vi "Engine Out - Port Fuel Injectors.vi"(0 "PFI Quantities [mg/inj]":sgl[](array[numeric]), 1 "PFI Timings [DBTDC]":sgl[](array[numeric]), 2 "BattV [V]":sgl, 5 "Control Inputs":T2={"Engine Speed [RPM]"=0.0, "Engine Status"=enum."STALLED", "Load Control \nMode"=enum."High-Idle Governor", "dt(s)"=0.0, "Number of Cylinders"=0, "Engine Displacement [cc]"=0.0, "StoichAFR"=0.0, "Q.LHV Fuel [kJ/kg]"=0.0, "BattV PSU [V]"=0.0, "12V PSU [V]"=0.0, "5V PSU [V]"=0.0, "Pedal Position [%]"=0.0, "Oil Pressure [kPa]"=0.0, "Oil Temp [C]"=0.0, "Oil Level [%]"=0.0, "Engine Coolant Temp (ECT) [C]"=0.0, "Engine Coolant Pressure [kPa]"=0.0, "Rail Pressure [bar]"=0.0, "Fuel Pressure [kPa]"=0.0, "Fuel Temp [C]"=0.0, "Vacuum Pressure [kPa]"=0.0, "Throttle Position [%]"=0.0, "Cam1 Advance [CAD]"=0.0, "Cam2 Advance [CAD]"=0.0, "Cam3 Advance [CAD]"=0.0, "Cam4 Advance [CAD]"=0.0, "CA50 Control Output [CAD]"=[], "CA50 Control Output Valid"=[], "Intake Air Temp (IAT) [C]"=0.0, "Barometric Air Pressure [kPa]"=0.0, "Intake Air Rel. Humidity [%]"=0.0, "Mass Air Flow (MAF) [kg/hr]"=0.0, "Turbo Inlet Air Pressure [kPa]"=0.0, "Turbo Inlet Air Temp [C]"=0.0, "Turbo Outlet Air Pressure [kPa]"=0.0, "Turbo Outlet Air Temp [C]"=0.0, "CAC Outlet Pressure [kPa]"=0.0, "CAC Outlet Temp [C]"=0.0, "Intake Manifold Pressure (MAP) [kPa]"=0.0, "Intake Manifold Temp (MAT) [C]"=0.0, "Exhaust Manifold Pressure [kPa]"=0.0, "Exhaust Manifold Temp [C]"=0.0, "HighP EGR Cooler Outlet Pressure [kPa]"=0.0, "HighP EGR Cooler Outlet Temp [C]"=0.0, "HighP EGR Differential Pressure [kPa]"=0.0, "HighP EGR Valve Position [%]"=0.0, "Turbo Outlet Exhaust Pressure [kPa]"=0.0, "Turbo Outlet Exhaust Temp [C]"=0.0, "VGT Position 1 [%]"=0.0, "VGT Position 2 [%]"=0.0, "Turbo Speed 1 [RPM]"=0.0, "Turbo Speed 2 [RPM]"=0.0, "LowP EGR Differential Pressure [kPa]"=0.0, "LowP EGR Valve Position [%]"=0.0, "UEGO1Lambda"=0.0, "UEGO1_Hot"=FALSE, "UEGO2Lambda"=0.0, "UEGO2_Hot"=FALSE, "Knock Intensity"=[], "Knock"=[]} {"Knock Intensity" format="%.2f"; "CA50 Control Output [CAD]" format="%.2f"; "Exhaust Manifold Temp [C]" format="%#_6f"; "UEGO2Lambda" format="%.2f"; "Intake Manifold Temp (MAT) [C]" format="%#_6f"; "UEGO1Lambda" format="%.2f"}) -> (11 "Injector 8":T1, 13 "Injector 7":T1, 14 "Injector 1":T1, 15 "Injector 2":T1, 16 "Injector 3":T1, 17 "Injector 4":T1, 18 "Injector 5":T1, 19 "Injector 6":T1)   [LabVIEW 2015, in "ECS-RT.lvlib"]
uses:
  ECS-RT.lvlib
  Typedefs/Control Inputs/Control Inputs.ctl
  Typedefs/EPT/Engine Status.ctl
  Typedefs/MISC/Load Control Mode.ctl
  Typedefs/Raw Outputs/PFI.ctl
  ECS-Shared.lvlib
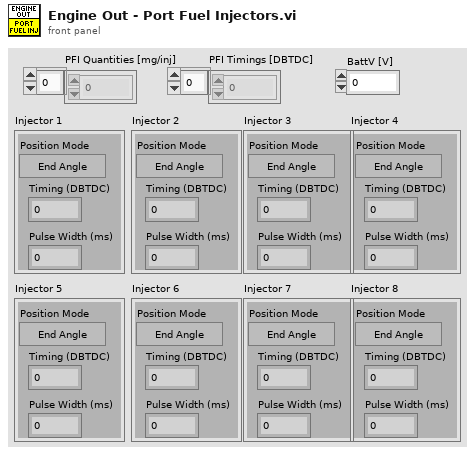
[diagram p1: front panel]
types:
  T1 = typedef "ECS-Shared.lvlib/PFI.ctl" = cluster{"Position Mode":bool, "Timing (DBTDC)":sgl, "Pulse Width (ms)":sgl}
  T2 = typedef "ECS-Shared.lvlib/Control Inputs.ctl" = cluster{"Engine Speed [RPM]":sgl, "Engine Status":T3, "Load Control \nMode":T4, "dt(s)":sgl, "Number of Cylinders":u8, "Engine Displacement [cc]":sgl, "StoichAFR":sgl, "Q.LHV Fuel [kJ/kg]":sgl, "BattV PSU [V]":sgl, "12V PSU [V]":sgl, "5V PSU [V]":sgl, "Pedal Position [%]":sgl, "Oil Pressure [kPa]":sgl, "Oil Temp [C]":sgl, "Oil Level [%]":sgl, "Engine Coolant Temp (ECT) [C]":sgl, "Engine Coolant Pressure [kPa]":sgl, "Rail Pressure [bar]":sgl, "Fuel Pressure [kPa]":sgl, "Fuel Temp [C]":sgl, "Vacuum Pressure [kPa]":sgl, "Throttle Position [%]":sgl, "Cam1 Advance [CAD]":sgl, "Cam2 Advance [CAD]":sgl, "Cam3 Advance [CAD]":sgl, "Cam4 Advance [CAD]":sgl, "CA50 Control Output [CAD]":sgl[], "CA50 Control Output Valid":bool[], "Intake Air Temp (IAT) [C]":sgl, "Barometric Air Pressure [kPa]":sgl, "Intake Air Rel. Humidity [%]":sgl, "Mass Air Flow (MAF) [kg/hr]":sgl, "Turbo Inlet Air Pressure [kPa]":sgl, "Turbo Inlet Air Temp [C]":sgl, "Turbo Outlet Air Pressure [kPa]":sgl, "Turbo Outlet Air Temp [C]":sgl, "CAC Outlet Pressure [kPa]":sgl, "CAC Outlet Temp [C]":sgl, "Intake Manifold Pressure (MAP) [kPa]":sgl, "Intake Manifold Temp (MAT) [C]":sgl, "Exhaust Manifold Pressure [kPa]":sgl, "Exhaust Manifold Temp [C]":sgl, "HighP EGR Cooler Outlet Pressure [kPa]":sgl, "HighP EGR Cooler Outlet Temp [C]":sgl, "HighP EGR Differential Pressure [kPa]":sgl, "HighP EGR Valve Position [%]":sgl, "Turbo Outlet Exhaust Pressure [kPa]":sgl, "Turbo Outlet Exhaust Temp [C]":sgl, "VGT Position 1 [%]":sgl, "VGT Position 2 [%]":sgl, "Turbo Speed 1 [RPM]":sgl, "Turbo Speed 2 [RPM]":sgl, "LowP EGR Differential Pressure [kPa]":sgl, "LowP EGR Valve Position [%]":sgl, "UEGO1Lambda":sgl, "UEGO1_Hot":bool, "UEGO2Lambda":sgl, "UEGO2_Hot":bool, "Knock Intensity":sgl[], "Knock":bool[]}
  T3 = typedef "ECS-Shared.lvlib/Engine Status.ctl" = enum16{"OFF", "STALLED", "CRANKING", "RUNNING", "ACCEL", "DECEL", "SAFE"}
  T4 = typedef "ECS-Shared.lvlib/Load Control Mode.ctl" = enum16{"No Governor", "Low-Idle Governor", "High-Idle Governor"}
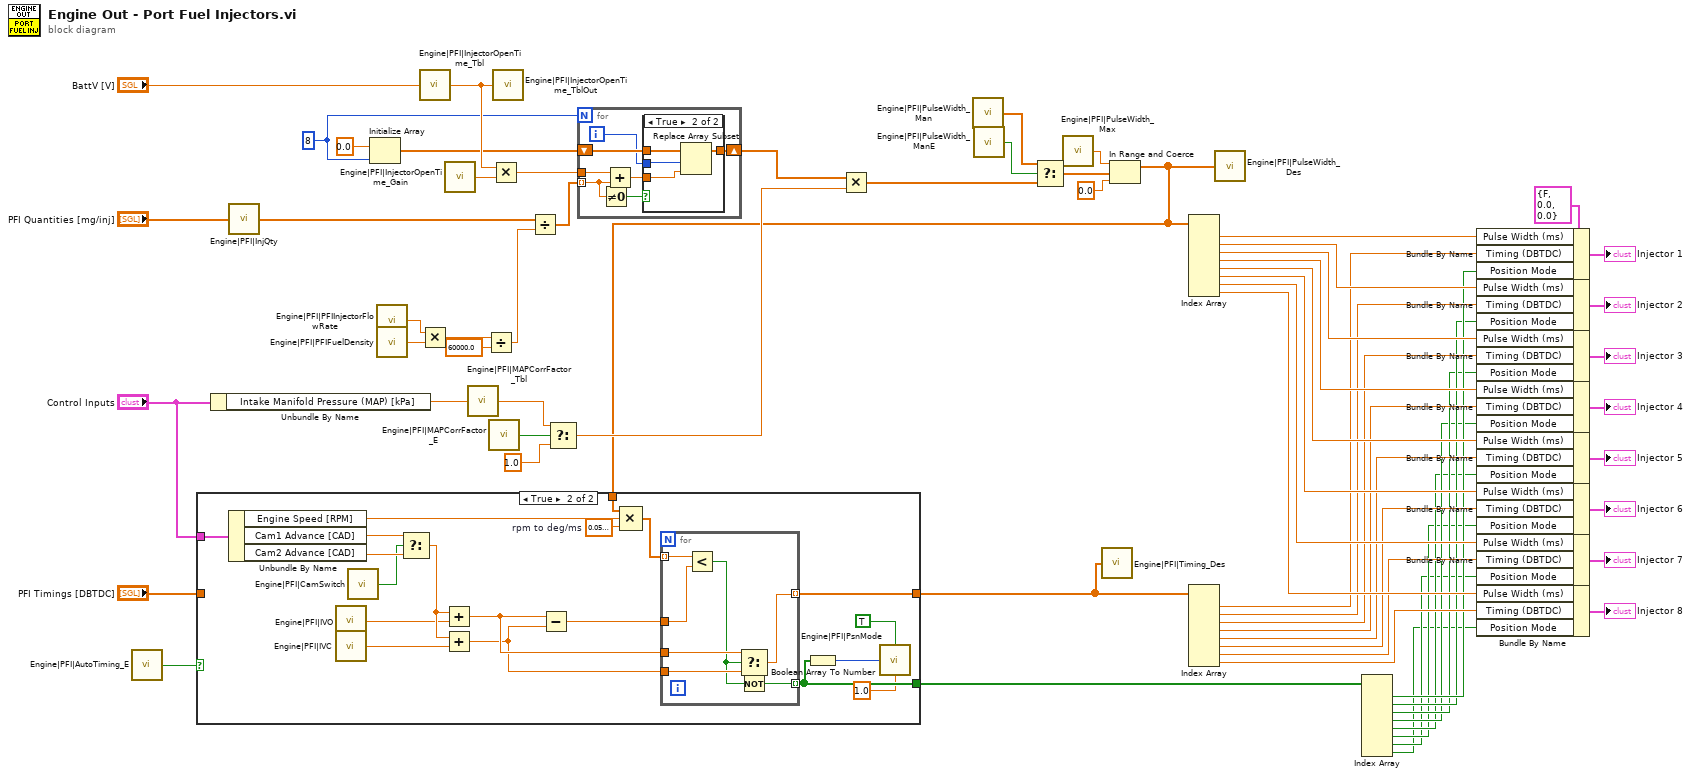
[diagram p0: block diagram]
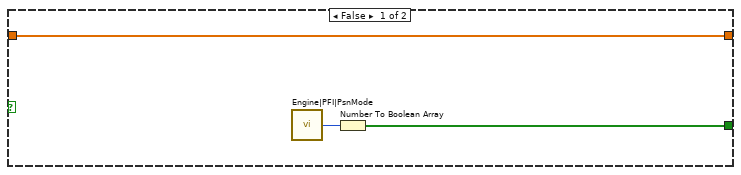
[diagram p3: hidden frame]
diagram:
  w1 = 8 ("dimension size")
  w43 = T1 {"Position Mode"=FALSE, "Timing (DBTDC)"=0.0, "Pulse Width (ms)"=0.0} ("Injector")
  n1 = call "Engine|PFI|AutoTiming_E"() -> ("Value"=w11:bool)
  n2 = Unbundle By Name("Control Inputs") -> ("Intake Manifold Pressure (MAP) [kPa]"=w46:sgl)
  n3 = call "Engine|PFI|InjQty"("Value"="PFI Quantities [mg/inj]") -> ()
  n4 = Initialize Array(sgl 0.0 ("t"), w1) -> (w3:sgl[])
  n5 = call "Engine|PFI|PFIInjectorFlowRate"() -> ("Value"=w64:sgl)
  n6 = call "Engine|PFI|PFIFuelDensity"() -> ("Value"=w65:sgl)
  n7 = call "Engine|PFI|InjectorOpenTime_Tbl"("X Index"="BattV [V]") -> ("Y"=w57:sgl)
  n8 = Multiply(x=w64, y=w65) -> (x*y=w60:sgl)
  n9 = call "Engine|PFI|InjectorOpenTime_Gain"() -> ("Value"=w63:sgl)
  n10 = call "Engine|PFI|MAPCorrFactor_Tbl"("X Index"=w46) -> ("Y"=w50:sgl)
  n11 = Divide(x=w60, y=sgl 60000.0) -> (x/y=w59:sgl)
  n12 = call "Engine|PFI|MAPCorrFactor_E"() -> ("Value"=w51:bool)
  n13 = Multiply(x=w57, y=w63) -> (x*y=w62:sgl)
  n14 = call "Engine|PFI|InjectorOpenTime_TblOut"("Value"=w57) -> ()
  n15 = Divide(x="PFI Quantities [mg/inj]", y=w59) -> (x/y=w61:sgl[])
  n16 = Select(t=w50, s=w51, f=sgl 1.0) -> (s? t:f=w48:sgl)
  n17 = for {
    N: w1 -> [_]
    tunnel: w62 -> [w72]
    tunnel: w61 -> [w69] mode=indexing
    shift-right: [w70] -> w2
    shift-left: w3 -> [w71]
    i -> [w66]
    n18 = Not Equal To 0?(x=w69) -> (x != 0?=w67:bool)
    n19 = Add(x=w72, y=w69) -> (x+y=w68:sgl)
    n20 = case shown="True" w67 {
      tunnel: w71 -> [w73 w77]
      tunnel: [w73 w76] -> w70
      tunnel: w66 -> [_ w75]
      tunnel: w68 -> [_ w74]
      frame False {
      }
      frame True {
        n21 = Replace Array Subset(array=w77, new element=w74, index=w75) -> (w76:sgl[])
      }
    }
  }
  n22 = Multiply(x=w2, y=w48) -> (x*y=w47:sgl[])
  n23 = call "Engine|PFI|PulseWidth_Man"() -> ("Value"=w53:sgl[])
  n24 = call "Engine|PFI|PulseWidth_ManE"() -> ("Value"=w54:bool)
  n25 = Select(t=w53, s=w54, f=w47) -> (s? t:f=w52:sgl[])
  n26 = call "Engine|PFI|PulseWidth_Max"() -> ("Value"=w56:sgl)
  n27 = In Range and Coerce(upper limit=w56, x=w52, lower limit=sgl 0.0 ("Value")) -> (coerced(x)=w8:sgl[])  [unwired: 1 out]
  n28 = case shown="True" w11 {
    tunnel: "PFI Timings [DBTDC]" -> [w80 _]
    tunnel: [w80 w90] -> w7
    tunnel: [w78 w84] -> w9
    tunnel: "Control Inputs" -> [_ w99]
    tunnel: w8 -> [_ w93]
    frame False {
      n29 = call "Engine|PFI|PsnMode"() -> ("Value"=w79:u8)
      n30 = Number To Boolean Array(number=w79) -> (Boolean array=w78:bool[])
    }
    frame True {
      w94 = sgl 0.06  # rpm to deg/ms
      n31 = Unbundle By Name(w99) -> ("Engine Speed [RPM]"=w95:sgl, "Cam1 Advance [CAD]"=w98:sgl, "Cam2 Advance [CAD]"=w97:sgl)
      n32 = call "Engine|PFI|IVO"() -> ("Value"=w88:sgl)
      n33 = call "Engine|PFI|IVC"() -> ("Value"=w87:sgl)
      n34 = call "Engine|PFI|CamSwitch"() -> ("Value"=w96:bool)
      n35 = Select(t=w98, s=w96, f=w97) -> (s? t:f=w89:sgl)
      n36 = Add(x=w89, y=w88) -> (x+y=w86:sgl)
      n37 = Add(x=w89, y=w87) -> (x+y=w85:sgl)
      n38 = Subtract(x=w86, y=w85) -> (x-y=w91:sgl)
      n39 = Compound Arithmetic op=MULTIPLY(w93, w95, w94) -> (w92:sgl[])
      n40 = for {
        tunnel: w92 -> [w106] mode=indexing
        tunnel: w91 -> [w105]
        tunnel: w86 -> [w104]
        tunnel: w85 -> [w103]
        tunnel: [w102] -> w90 mode=indexing
        tunnel: [w100] -> w84 mode=indexing
        n41 = Less?(x=w106, y=w105) -> (x < y?=w101:bool)
        n42 = Select(t=w104, s=w101, f=w103) -> (s? t:f=w102:sgl)
        n43 = Not(x=w101) -> (.not. x?=w100:bool)
      }
      n44 = Boolean Array To Number(Boolean array=w84) -> (number=w83:u32)
      n45 = call "Engine|PFI|PsnMode"("%/100"=sgl 1.0, "Value"=w83, "Adapt"=TRUE) -> ()
    }
  }
  n46 = call "Engine|PFI|Timing_Des"("Value"=w7) -> ()
  n47 = Index Array(array=w8) -> (element #1=w36:sgl, element #2=w35:sgl, element #3=w34:sgl, element #4=w33:sgl, element #5=w32:sgl, element #6=w31:sgl, element #7=w30:sgl, element #8=w29:sgl)  [unwired: 8 in]
  n48 = Index Array(array=w7) -> (element #1=w28:sgl, element #2=w27:sgl, element #3=w26:sgl, element #4=w25:sgl, element #5=w24:sgl, element #6=w23:sgl, element #7=w22:sgl, element #8=w21:sgl)  [unwired: 8 in]
  n49 = call "Engine|PFI|PulseWidth_Des"("Value"=w8) -> ()
  n50 = Index Array(array=w9) -> (element #1=w19:bool, element #2=w18:bool, element #3=w17:bool, element #4=w16:bool, element #5=w15:bool, element #6=w14:bool, element #7=w13:bool, element #8=w12:bool)  [unwired: 8 in]
  n51 = Bundle By Name(cluster=w43, "Pulse Width (ms)"=w36, "Timing (DBTDC)"=w28, "Position Mode"=w19) -> (→"Injector 1":T1)
  n52 = Bundle By Name(cluster=w43, "Pulse Width (ms)"=w35, "Timing (DBTDC)"=w27, "Position Mode"=w18) -> (→"Injector 2":T1)
  n53 = Bundle By Name(cluster=w43, "Pulse Width (ms)"=w34, "Timing (DBTDC)"=w26, "Position Mode"=w17) -> (→"Injector 3":T1)
  n54 = Bundle By Name(cluster=w43, "Pulse Width (ms)"=w33, "Timing (DBTDC)"=w25, "Position Mode"=w16) -> (→"Injector 4":T1)
  n55 = Bundle By Name(cluster=w43, "Pulse Width (ms)"=w32, "Timing (DBTDC)"=w24, "Position Mode"=w15) -> (→"Injector 5":T1)
  n56 = Bundle By Name(cluster=w43, "Pulse Width (ms)"=w31, "Timing (DBTDC)"=w23, "Position Mode"=w14) -> (→"Injector 6":T1)
  n57 = Bundle By Name(cluster=w43, "Pulse Width (ms)"=w30, "Timing (DBTDC)"=w22, "Position Mode"=w13) -> (→"Injector 7":T1)
  n58 = Bundle By Name(cluster=w43, "Pulse Width (ms)"=w29, "Timing (DBTDC)"=w21, "Position Mode"=w12) -> (→"Injector 8":T1)
